vi "ziQualifyPath.vi"(2 "Path In":string, 3 "Handle In":T1 {"Handle" format="0x%08x"; "Conn" format="0x%08x"}) -> (0 "Path Out":string, 1 "Handle Out":T1 {"Handle" format="0x%08x"; "Conn" format="0x%08x"})   [LabVIEW 2009, in "Zurich Instruments LabOne.lvlib"]
uses:
  <instrlib>/Zurich Instruments LabOne/Zurich Instruments LabOne.lvlib
  <instrlib>/Zurich Instruments LabOne/Public/ziTypeHandle.ctl
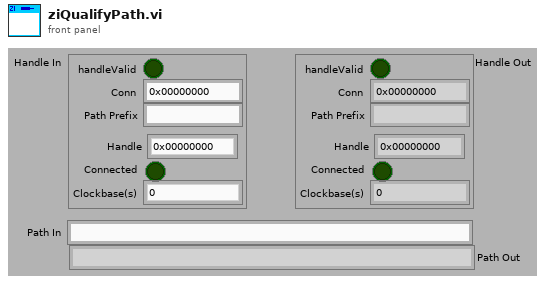
[diagram p1: front panel]
types:
  T1 = typedef "Zurich Instruments LabOne.lvlib/ziTypeHandle.ctl" = cluster{"handleValid":bool, "Conn":u64, "Path Prefix":string, "Handle":u64, "Connected":bool, "Clockbase(s)":dbl}
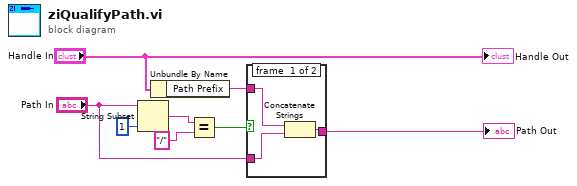
[diagram p0: block diagram]
diagram:
  n1 = String Subset(string="Path In", length (rest)=1 ("length (rest)")) -> (substring=w6:string)  [unwired: 1 out]
  n2 = Unbundle By Name("Handle In") -> ("Path Prefix"=w3:string)
  n3 = Equal?(x=w6, y="/") -> (x = y?=w8:bool)
  n4 = case shown="False" w8 {
    tunnel: w3 -> [w9 _]
    tunnel: [w11 w12] -> w4
    tunnel: "Path In" -> [w10 w12]
    frame #0 {
      n5 = Concatenate Strings(w9, w10) -> (w11:string)
    }
    frame #1 {
    }
  }
  "Path Out" <- w4
  "Handle Out" <- "Handle In"
